vi "AllyAreaObstacle.vi"(0 "Robot":refnum<class "Robot.lvclass">, 2 "Game":refnum<class "Game.lvclass">, 4 "ArrayOfObstacles in":T1[](array[typedef]), 7 "influence radius":dbl, 11 "multiplier":dbl) -> (18 "ArrayOfObstacles out":T1[](array[typedef]))   [LabVIEW 2023, in "Robot.lvclass"]
uses:
  Robot.lvclass
  C:/Users/lucio/Desktop/roboime/SSL_AI/Object_class/Object.lvclass
  obstacle.ctl
  Game_class/Game.lvclass
  Game_class/Game.lvclass/Game.ctl
  Object_class/Object.lvclass/Object.ctl
  Field_class/Field.lvclass/Field.ctl
  Field_class/Read ourGoalPosition.vi
  Object_class/Read position(x,y).vi
  Game_class/Read FieldRef.vi
  <vilib>/Analysis/1siggen.llb/Ramp Pattern by Delta.vi
  Field_class/Field.lvclass
  <vilib>/Analysis/NI_AALBase.lvlib
  Utilities_class/Utilities.lvclass
panel:
  out "object out":refnum<class "Robot.lvclass">
  in  "object in":refnum<class "Robot.lvclass">
  out "error out":errorcluster
  in  "error in (no error)":errorcluster
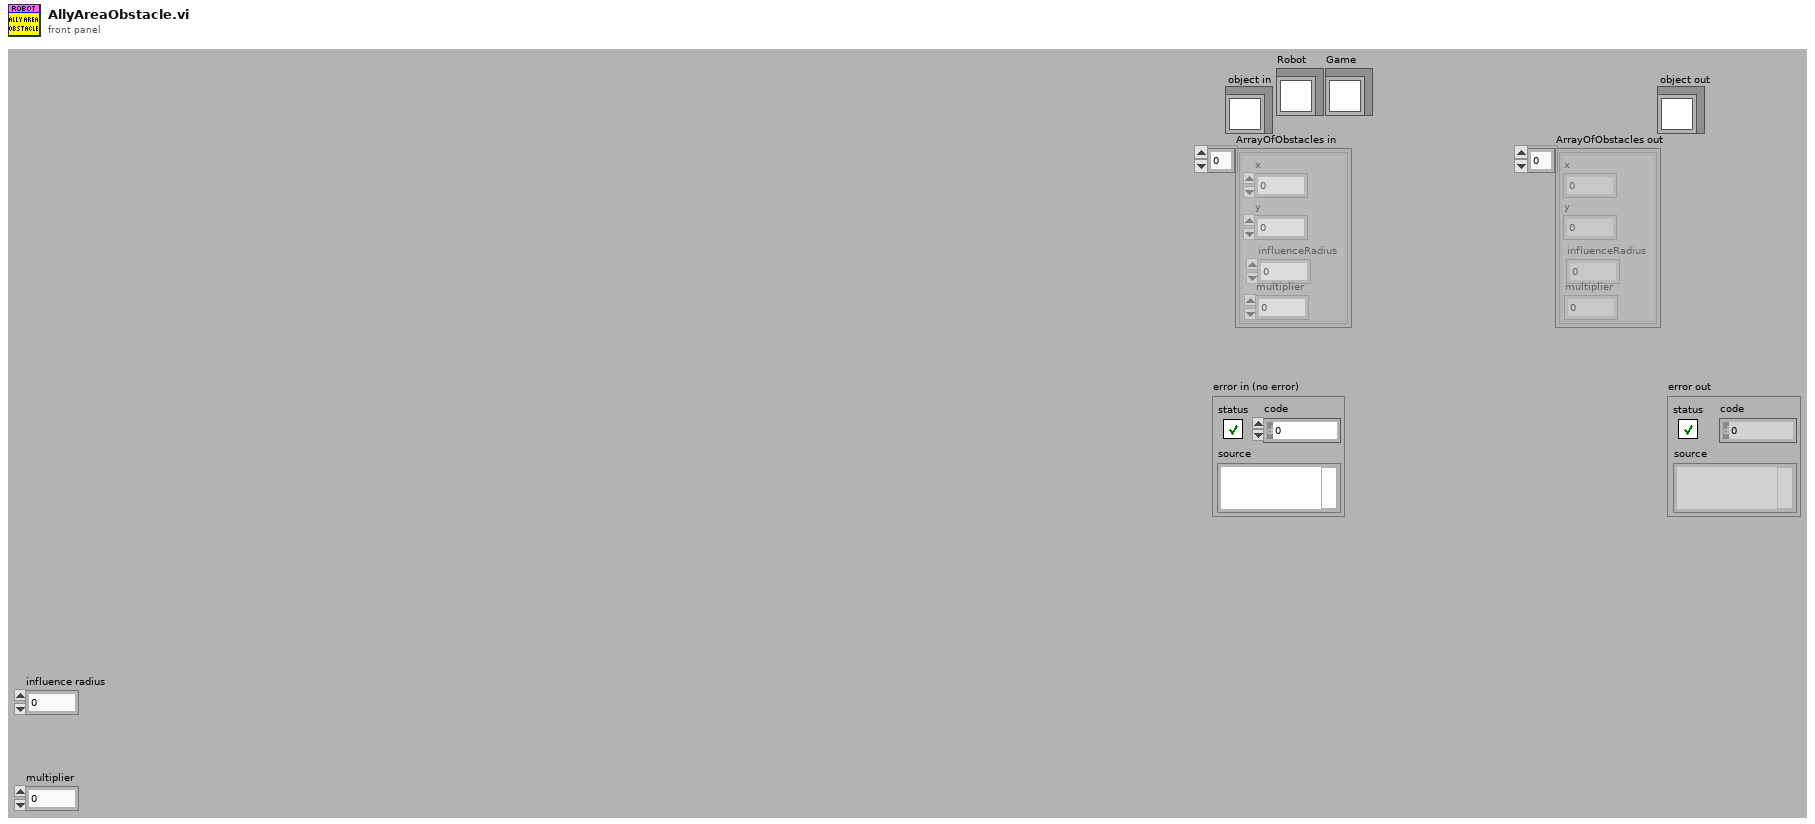
[diagram p1: front panel]
types:
  T1 = typedef "obstacle.ctl" = cluster{"x":dbl, "y":dbl, "influenceRadius":dbl, "multiplier":dbl}
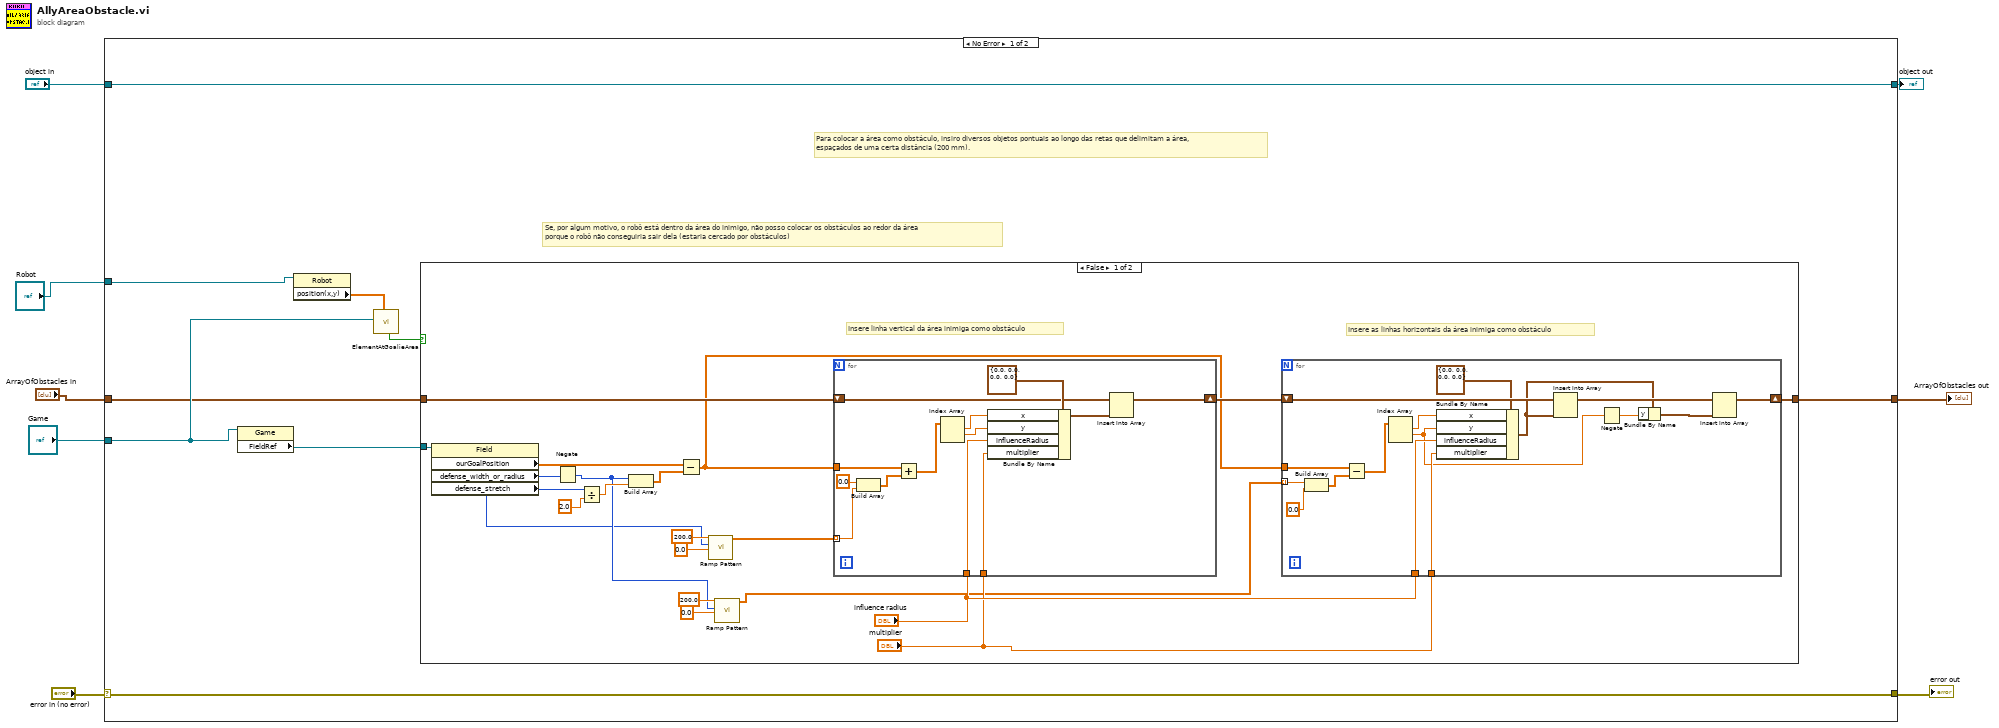
[diagram p0: block diagram]
diagram:
  n1 = case shown="No Error" "error in (no error)" {
    selector: "error in (no error)" -> [w16 w69]
    tunnel: [w16 w69] -> w7
    tunnel: [w17 w68] -> w5
    tunnel: "object in" -> [w17 w68]
    tunnel: [w12 _] -> w4
    tunnel: "Game" -> [w11 _]
    tunnel: "Robot" -> [w10 _]
    tunnel: "ArrayOfObstacles in" -> [w9 _]
    frame No Error {
      # "Para colocar a área como obstáculo, insiro diversos objetos pontuais ao longo das retas que delimitam a área,\nespaçados de uma certa distância (200 mm)."
      # "Se, por algum motivo, o robô está dentro da área do inimigo, não posso colocar os obstáculos ao redor da área\nporque o robô não conseguiria sair dela (estaria cercado por obstáculos)"
      n2 = property class="Game"(reference=w11) -> ("FieldRef"=w13:refnum<class "Field.lvclass">)  [unwired: 1 in, 2 out]
      n3 = property class="Robot"(reference=w10) -> ("position(x,y)"=w15:dbl[])  [unwired: 1 in, 2 out]
      n4 = call "ElementAtGoalieArea.vi"("Elemento pos."=w15, "Game"=w11) -> ("Element at enemy goalkeeper area?"=w14:bool)  [unwired: 5 in, 4 out]
      n5 = case shown="False" w14 {
        tunnel: w13 -> [w37 _]
        tunnel: w9 -> [w30 w67]
        tunnel: [w28 w67] -> w12
        frame False {
          # "Insere as linhas horizontais da área inimiga como obstáculo"
          # "Insere linha vertical da área inimiga como obstáculo"
          n6 = property class="Field"(reference=w37) -> ("ourGoalPosition"=w22:dbl[], "defense_width_or_radius"=w20:i32, "defense_stretch"=w18:i32)  [unwired: 1 in, 2 out]
          n7 = Negate(x=w20) -> (-x=w19:i32)
          n8 = Divide(x=w18, y=2.0) -> (x/y=w34:dbl)
          n9 = Build Array(w19, w34) -> (w36:dbl[])
          n10 = Subtract(x=w22, y=w36) -> (x-y=w21:dbl[])
          n11 = call-poly <vilib>:"Ramp Pattern.vi"("start"=0.0, "end"=w18, "delta"=200.0) -> ("Ramp Pattern"=w31:dbl[])  [unwired: 6 in, 2 out]
          n12 = call-poly <vilib>:"Ramp Pattern.vi"("start"=0.0, "end"=w19, "delta"=200.0) -> ("Ramp Pattern"=w23:dbl[])  [unwired: 6 in, 2 out]
          n13 = for {
            tunnel: w31 -> [w59] mode=indexing
            shift-right: [w64] -> w29
            shift-left: w30 -> [w63]
            tunnel: "influence radius" -> [w55]
            tunnel: "multiplier" -> [w54]
            tunnel: w21 -> [w62]
            n14 = Build Array(0.0 ("element"), w59) -> (w61:dbl[])
            n15 = Add(x=w62, y=w61) -> (x+y=w56:dbl[])
            n16 = Index Array(array=w56) -> (element #1=w58:dbl, element #2=w57:dbl)  [unwired: 2 in]
            n17 = Bundle By Name(cluster=T1 {"x"=0.0, "y"=0.0, "influenceRadius"=0.0, "multiplier"=0.0} ("ArrayOfObstacles in 2"), "x"=w58, "y"=w57, "influenceRadius"=w55, "multiplier"=w54) -> (w65:T1)
            n18 = Insert Into Array(array=w63, new element=w65) -> (w64:T1[])  [unwired: 1 in]
          }
          n19 = for {
            shift-right: [w44] -> w28
            shift-left: w29 -> [w53]
            tunnel: "influence radius" -> [w41]
            tunnel: "multiplier" -> [w48]
            tunnel: w23 -> [w46] mode=indexing
            tunnel: w21 -> [w52]
            n20 = Build Array(w46, 0.0 ("element")) -> (w51:dbl[])
            n21 = Subtract(x=w52, y=w51) -> (x-y=w49:dbl[])
            n22 = Index Array(array=w49) -> (element #1=w50:dbl, element #2=w38:dbl)  [unwired: 2 in]
            n23 = Bundle By Name(cluster=T1 {"x"=0.0, "y"=0.0, "influenceRadius"=0.0, "multiplier"=0.0} ("ArrayOfObstacles in 2"), "x"=w50, "y"=w38, "influenceRadius"=w41, "multiplier"=w48) -> (w40:T1)
            n24 = Insert Into Array(array=w53, new element=w40) -> (w45:T1[])  [unwired: 1 in]
            n25 = Negate(x=w38) -> (-x=w39:dbl)
            n26 = Bundle By Name(cluster=w40, "y"=w39) -> (w42:T1)
            n27 = Insert Into Array(array=w45, new element=w42) -> (w44:T1[])  [unwired: 1 in]
          }
        }
        frame True {
        }
      }
    }
    frame Error {
    }
  }
  "error out" <- w7
  "object out" <- w5
  "ArrayOfObstacles out" <- w4
